vi "Emergency Stop.vi"(0 "ESTOP References":T1) -> ()   [LabVIEW 2017]
uses:
  C:/Program Files/National Instruments/LabVIEW 2017/user.lib/aerotech/2010/Bin/Aerotech.A3200.dll
  Program Files/National Instruments/LabVIEW 2017/user.lib/aerotech/2010/Bin/Aerotech.A3200.dll
  <vilib>/DAQmx/write.llb/DAQmx Write (Digital Bool 1Line 1Point).vi
  <vilib>/DAQmx/read.llb/DAQmx Read (Digital 1D Bool 1Chan 1Samp).vi
  <vilib>/DAQmx/write.llb/DAQmx Write (Digital 1D Bool 1Chan 1Samp).vi
  <vilib>/DAQmx/miscellaneous.llb/DAQmx Fill In Error Info.vi
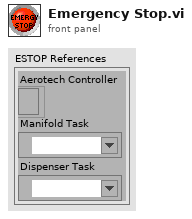
[diagram p1: front panel]
types:
  T1 = cluster{"Aerotech Controller":refnum<k24>, "Manifold Task":refnum<k21>, "Dispenser Task":refnum<k21>}
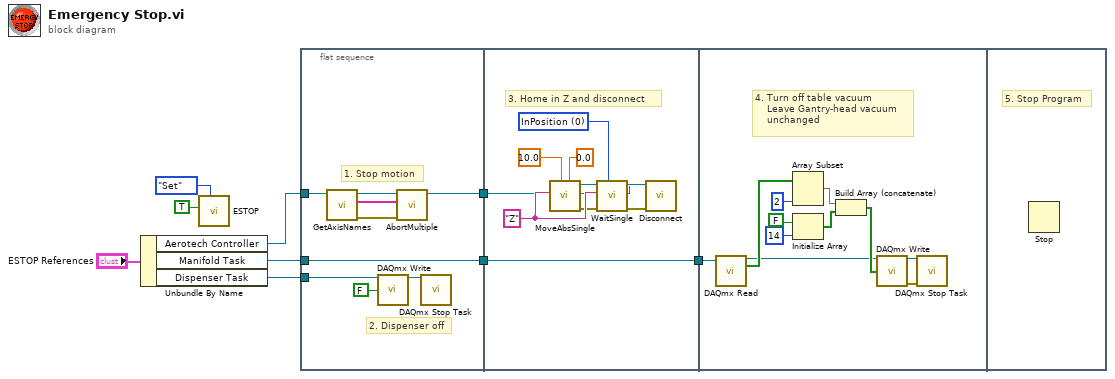
[diagram p0: block diagram]
diagram:
  n1 = Unbundle By Name("ESTOP References") -> ("Aerotech Controller"=w8:refnum<k24>, "Manifold Task"=w2:refnum<k21>, "Dispenser Task"=w1:refnum<k21>)
  n2 = call "ESTOP.vi"("Get/Set"=enum16{"Get", "Set"}."Set", "Value In"=TRUE) -> ()  [unwired: 9 in, 1 out]
  n3 = flat-sequence {
    tunnel: w1 -> [w18]
    tunnel: w8 -> [w16]
    tunnel: w2 -> [w11]
    tunnel: [w11] -> w5
    tunnel: [w10] -> w3
    tunnel: w5 -> [w28]
    tunnel: [w28] -> w4
    tunnel: w3 -> [w19]
    tunnel: w4 -> [w29]
    frame #0 {
      # "1. Stop motion"
      # "2. Dispenser off"
      n4 = call <userlib>:"GetAxisNames.vi"("controller in"=w16) -> ("error out"=w13:errorcluster, "axis names"=w14:string[], "controller out"=w15:refnum<k24>)  [unwired: 8 in]
      n5 = call-poly <vilib>:"DAQmx Write.vi"("task/channels in"=w18, "data"=FALSE) -> ("task out"=w12:refnum<k21>)  [unwired: 11 in, 2 out]
      n6 = call <userlib>:"AbortMultiple.vi"("error in (no error)"=w13, "axis names"=w14, "controller in"=w15) -> ("controller out"=w10:refnum<k24>)  [unwired: 7 in, 1 out]
      n7 = call <vilib>:"DAQmx Stop Task.vi"("task/channels in"=w12) -> ()  [unwired: 13 in, 2 out]
    }
    frame #1 {
      w27 = 0 items=["InPosition", "MoveDone"] ("wait option?")
      w25 = "Z" ("axis name")
      # "3. Home in Z and disconnect"
      n8 = call <userlib>:"MoveAbsSingle.vi"("position"=0.0, "speed"=10.0, "axis name"=w25, "controller in"=w19) -> ("error out"=w24:errorcluster, "controller out"=w22:refnum<k24>)  [unwired: 6 in]
      n9 = call <userlib>:"WaitSingle.vi"("wait option?"=w27, "error in (no error)"=w24, "axis name"=w25, "controller in"=w22) -> ("error out"=w26:errorcluster, "controller out"=w23:refnum<k24>)  [unwired: 5 in, 1 out]
      n10 = call <userlib>:"Disconnect.vi"("error in (no error)"=w26, "controller"=w23) -> ()  [unwired: 9 in, 1 out]
    }
    frame #2 {
      # "4. Turn off table vacuum\n    Leave Gantry-head vacuum\n    unchanged"
      n11 = call-poly <vilib>:"DAQmx Read.vi"("task/channels in"=w29) -> ("task out"=w32:refnum<k21>, "data"=w33:bool[])  [unwired: 12 in, 1 out]
      n12 = Array Subset(array=w33, length=2) -> (w35:bool[])  [unwired: 1 in]
      n13 = Initialize Array(FALSE ("Boolean"), 14 ("dimension size")) -> (w36:bool[])
      n14 = Build Array (concatenate)(w35, w36) -> (w37:bool[])
      n15 = call-poly <vilib>:"DAQmx Write.vi"("task/channels in"=w32, "data"=w37) -> ("task out"=w39:refnum<k21>, "error out"=w38:errorcluster)  [unwired: 11 in, 1 out]
      n16 = call <vilib>:"DAQmx Stop Task.vi"("task/channels in"=w39, "error in"=w38) -> ()  [unwired: 12 in, 2 out]
    }
    frame #3 {
      # "5. Stop Program"
      n17 = Stop() -> ()  [unwired: 1 in]
    }
  }
